vi "ultrasonicGlobal.vi"() -> ()   [LabVIEW 2014]
panel:
  in  "ultrasonicValue":dbl
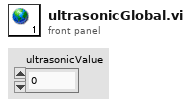
[diagram p1: front panel]
diagram:
